vi "1.4bis.vi"() -> ()   [LabVIEW 2013]
panel:
  out "Temperatura Convertida":dbl
  in  "Temperatura a Convertir":dbl
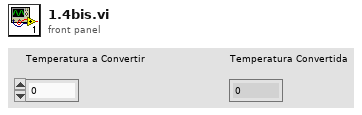
[diagram p1: front panel]
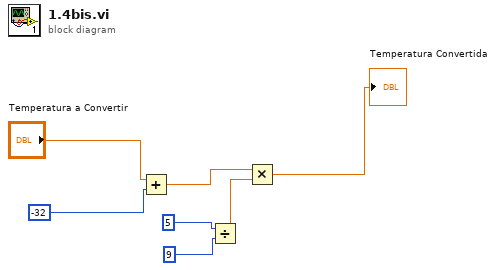
[diagram p0: block diagram]
diagram:
  n1 = Add(x="Temperatura a Convertir", y=-32) -> (x+y=w6:dbl)
  n2 = Divide(x=5, y=9) -> (x/y=w3:dbl)
  n3 = Multiply(x=w6, y=w3) -> (x*y=→"Temperatura Convertida":dbl)
